vi "sender_udp.vi"() -> ()   [LabVIEW 2022 SP3]
panel:
  in  "number":dbl
  in  "change to binary":bool
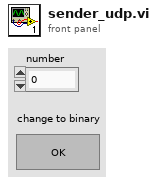
[diagram p1: front panel]
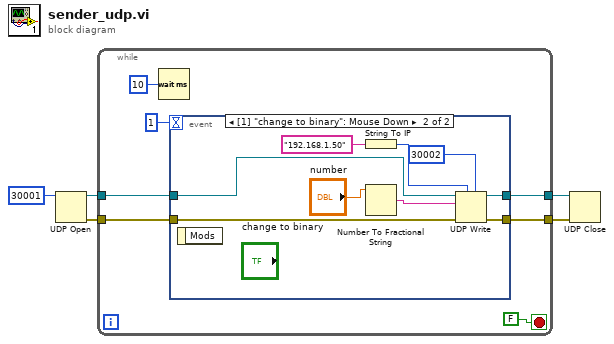
[diagram p0: block diagram]
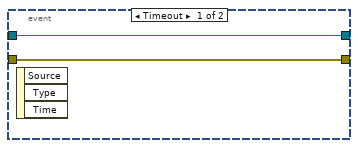
[diagram p2: hidden frame]
diagram:
  n1 = UDP Open(11:u16 30001 ("port")) -> (port=w4:refnum<k16>, 0:w1:errorcluster)  [unwired: 4 in, 1 out]
  n2 = while {
    tunnel: w4 -> [w10]
    tunnel: [w9] -> w3
    tunnel: [w8] -> w2
    tunnel: w1 -> [w6]
    stop <- FALSE stop-if-true
    n3 = Wait (ms)(milliseconds to wait=u32 10) -> ()  [unwired: 1 out]
    n4 = event shown="[1] \"change to binary\": Mouse Down" {
      selector: _ -> [_ _]
      dyn-events: _ -> [_ _]
      timeout: 1 -> [_ _]
      tunnel: w10 -> [w14 w19]
      tunnel: [w14 w21] -> w9
      tunnel: [w13 w20] -> w8
      tunnel: w6 -> [w13 w18]
      event Timeout {
        n5 = event-data() -> ()  [unwired: 1 in, 3 out]
      }
      event "change to binary": Mouse Down {
        n6 = event-data() -> ()  [unwired: 1 in, 1 out]
        n7 = String To IP(1:"192.168.1.50" ("name")) -> (0:w15:u32)
        n8 = Number To Fractional String(number="number") -> (F-format string=w22:string)  [unwired: 3 in]
        n9 = UDP Write(address=w15, port or service name=u16 30002, connection ID=w19, data in=w22, 8:w18) -> (error out=w20:errorcluster, 3:w21:refnum<k16>)  [unwired: 1 in]
      }
    }
  }
  n10 = UDP Close(connection ID=w3, 8:w2) -> ()  [unwired: 2 out]
